vi "Single wire operator.vi"(8 "error in (no error)":errorcluster, 9 "Operator matrix":T1, 10 "Wire in":T2, 11 "G-UE in":refnum<class "G-UE.lvclass">) -> (0 "error out":errorcluster, 3 "G-UE out":refnum<class "G-UE.lvclass">)   [LabVIEW 2016, in "G-UE.lvclass"]
uses:
  G-UE.lvclass
  TypeDefs/Circuit Cluster.ctl
  GateAbst/GateAbst.lvclass
  <vilib>/Analysis/Matrix/Datatypes/ComplexMatrix.ctl
  G-UE.lvclass/G-UE.ctl
  <vilib>/Analysis/7linalg.llb/Complex Kronecker Product.vi
  <vilib>/Analysis/baseanly.llb/Complex A x B.vi
  <vilib>/Analysis/Matrix/NI_Matrix.lvlib
  <vilib>/Analysis/NI_AALPro.lvlib
  <vilib>/Analysis/NI_AALBase.lvlib
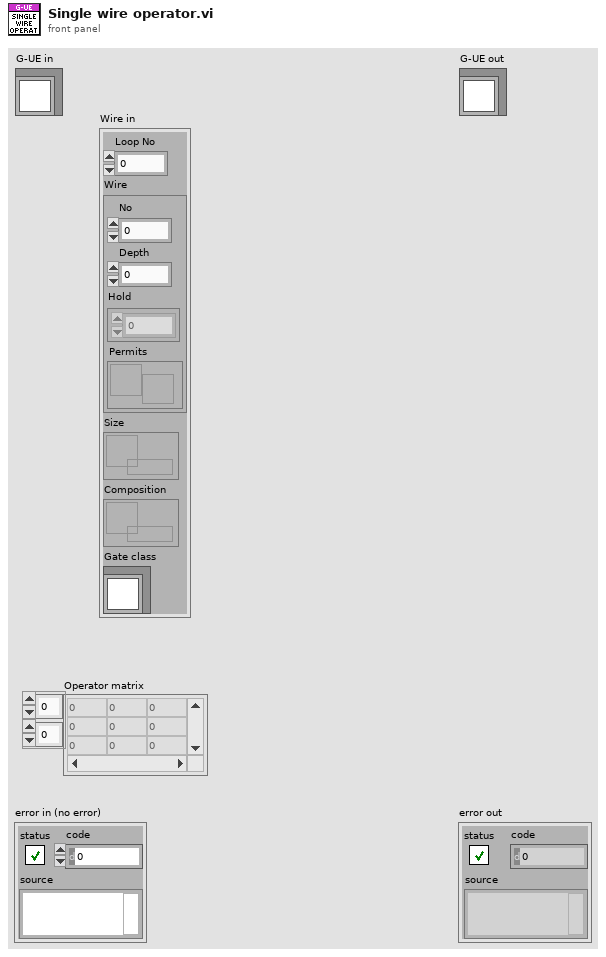
[diagram p1: front panel]
types:
  T1 = typedef "NI_Matrix.lvlib/ComplexMatrix.ctl" = cdb[][]
  T2 = typedef "Circuit Cluster.ctl" = cluster{"Loop No":i32, "Wire":cluster{"No":i32, "Depth":i32, "Hold":i32[][], "Permits":refnum<notifier>}, "Size":refnum<queue>, "Composition":refnum<queue>, "Gate class":refnum<class "GateAbst.lvclass">}
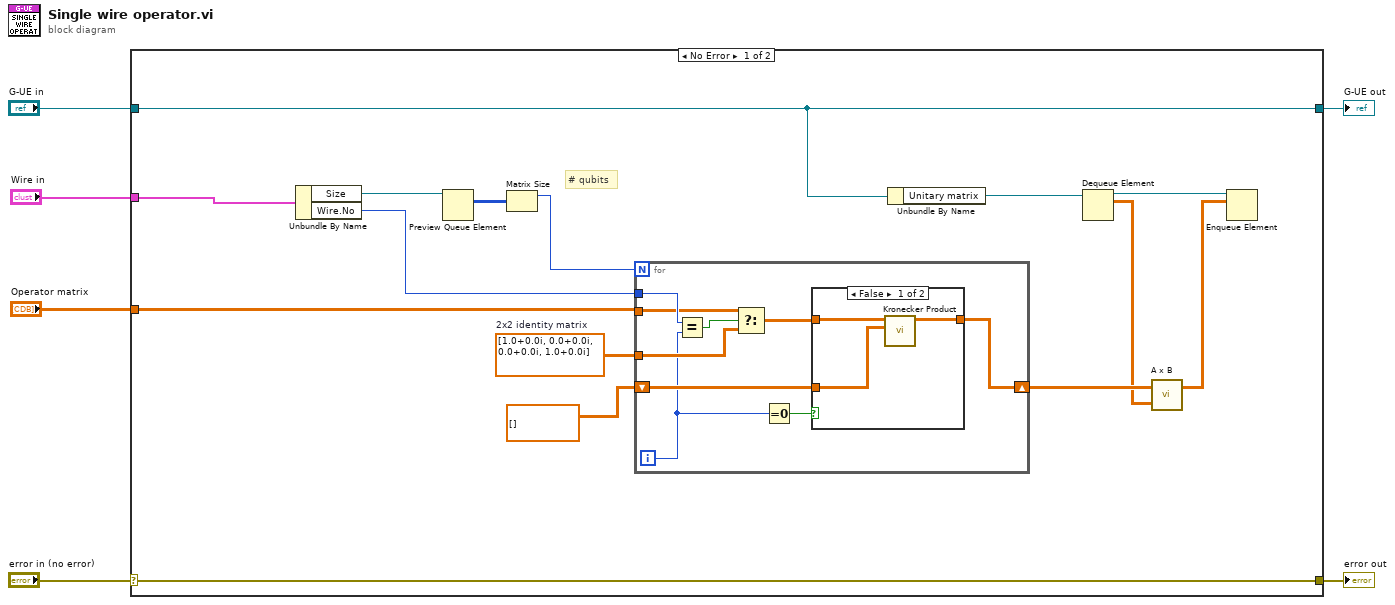
[diagram p0: block diagram]
diagram:
  n1 = case shown="No Error" "error in (no error)" {
    selector: "error in (no error)" -> [w21 w36]
    tunnel: [w21 w36] -> w5
    tunnel: [w17 w35] -> w3
    tunnel: "G-UE in" -> [w17 w35]
    tunnel: "Wire in" -> [w11 _]
    tunnel: "Operator matrix" -> [w10 _]
    frame No Error {
      w19 = T1 [[1.0+0.0i, 0.0+0.0i], [0.0+0.0i, 1.0+0.0i]]  # 2x2 identity matrix
      # "# qubits"
      n2 = Unbundle By Name(w11) -> ("Size"=w16:refnum<queue>, "Wire.No"=w20:i32)
      n3 = Preview Queue Element(queue=w16) -> (element=w8:i32[][])  [unwired: 2 in, 3 out]
      n4 = Matrix Size(0:w8) -> (1:w7:i32)  [unwired: 1 out]
      n5 = for {
        N: w7 -> [_]
        tunnel: w20 -> [w30]
        tunnel: w19 -> [w26]
        tunnel: w10 -> [w28]
        shift-right: [w27] -> w18
        shift-left: T1 [] ("State") -> [w25]
        i -> [w22]
        n6 = Equal?(x=w30, y=w22) -> (x = y?=w29:bool)
        n7 = Select(t=w28, s=w29, f=w26) -> (s? t:f=w24:T1)
        n8 = Equal To 0?(x=w22) -> (x = 0?=w23:bool)
        n9 = case shown="False" w23 {
          tunnel: [w33 w34] -> w27
          tunnel: w25 -> [w32 _]
          tunnel: w24 -> [w31 w34]
          frame False {
            n10 = call-poly <vilib>:"Kronecker Product.vi"("B"=w32, "A"=w31) -> ("Kronecker Product"=w33:T1)  [unwired: 8 in, 1 out]
          }
          frame True {
          }
        }
      }
      n11 = Unbundle By Name(w17) -> ("Unitary matrix"=w15:refnum<queue>)
      n12 = Dequeue Element(queue=w15) -> (queue out=w12:refnum<queue>, element=w14:T1)  [unwired: 2 in, 2 out]
      n13 = call-poly <vilib>:"A x B.vi"("B"=w14, "A"=w18) -> ("A x B"=w13:T1)  [unwired: 1 out]
      n14 = Enqueue Element(queue=w12, element=w13) -> ()  [unwired: 2 in, 3 out]
    }
    frame Error {
    }
  }
  "error out" <- w5
  "G-UE out" <- w3
